vi "Output.vi"(8 "error in (no error)":errorcluster, 10 "SignalGeneratorParameter":cluster{"Frequency":dbl, "Amplitude":dbl}={"Frequency"=10.0, "Amplitude"=1.0}, 11 "GenSin in":refnum<class "GenSquare.lvclass">) -> (0 "error out":errorcluster, 2 "Waveform":waveform(dbl), 3 "GenSin out":refnum<class "GenSquare.lvclass">)   [LabVIEW 2013, in "GenSquare.lvclass"]
uses:
  GenSquare.lvclass
  <vilib>/measure/NI_MABase.lvlib
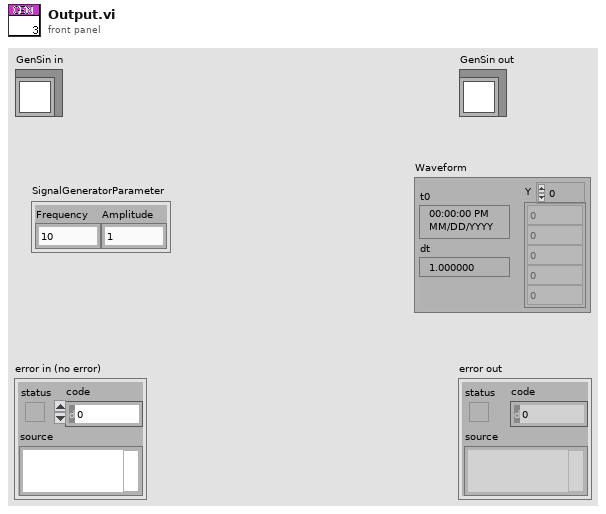
[diagram p1: front panel]
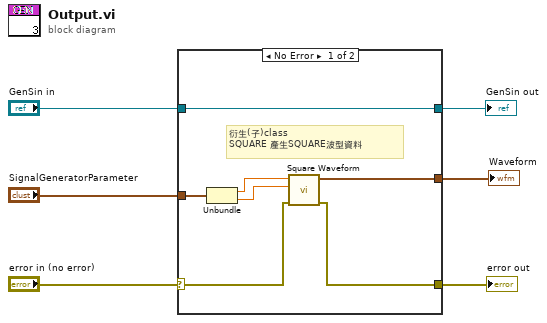
[diagram p0: block diagram]
diagram:
  n1 = case shown="No Error" "error in (no error)" {
    selector: "error in (no error)" -> [w9 w15]
    tunnel: [w8 w15] -> w2
    tunnel: [w13 w14] -> w5
    tunnel: "GenSin in" -> [w13 w14]
    tunnel: "SignalGeneratorParameter" -> [w12 _]
    tunnel: [w7 _] -> w1
    frame No Error {
      # "衍生(子)class\nSQUARE 產生SQUARE波型資料"
      n2 = Unbundle(w12) -> ("Frequency"=w11:dbl, "Amplitude"=w10:dbl)
      n3 = call <vilib>:"Square Waveform.vi"("error in (no error)"=w9, "amplitude"=w10, "frequency"=w11) -> ("error out"=w8:errorcluster, "signal out"=w7:waveform(dbl))  [unwired: 7 in]
    }
    frame Error {
    }
  }
  "error out" <- w2
  "GenSin out" <- w5
  "Waveform" <- w1
